vi "Remove.vi"(8 "error in (no error)":errorcluster, 10 "BrowerComponentIDs(\"\")":string[](array[string]), 11 "reference in":refnum<class "BrowerComponent.lvclass">) -> (0 "error out":errorcluster, 3 "reference out":refnum<class "BrowerComponent.lvclass">)   [LabVIEW 2015, in "BrowerComponent.lvclass"]
uses:
  BrowerComponent.lvclass
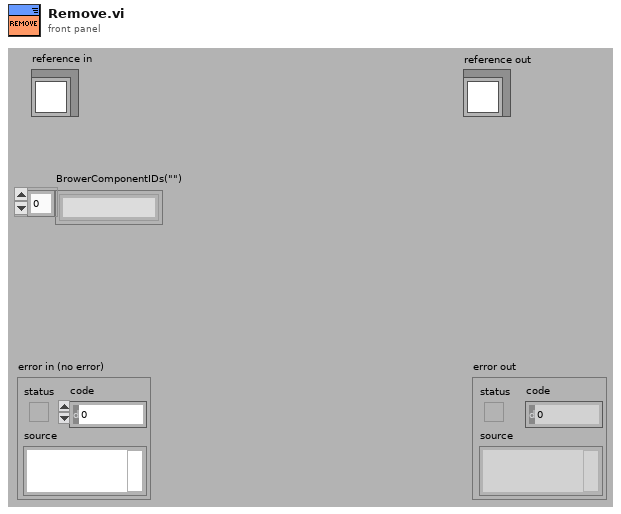
[diagram p1: front panel]
types:
  T1 = typedef "BrowerComponent.lvclass/ObjectAttributes.ctl" = cluster{"ComponentID":string, "SymbolIndex":i32, "ComponentName":string, "PartsOfComponent_dict":variant}
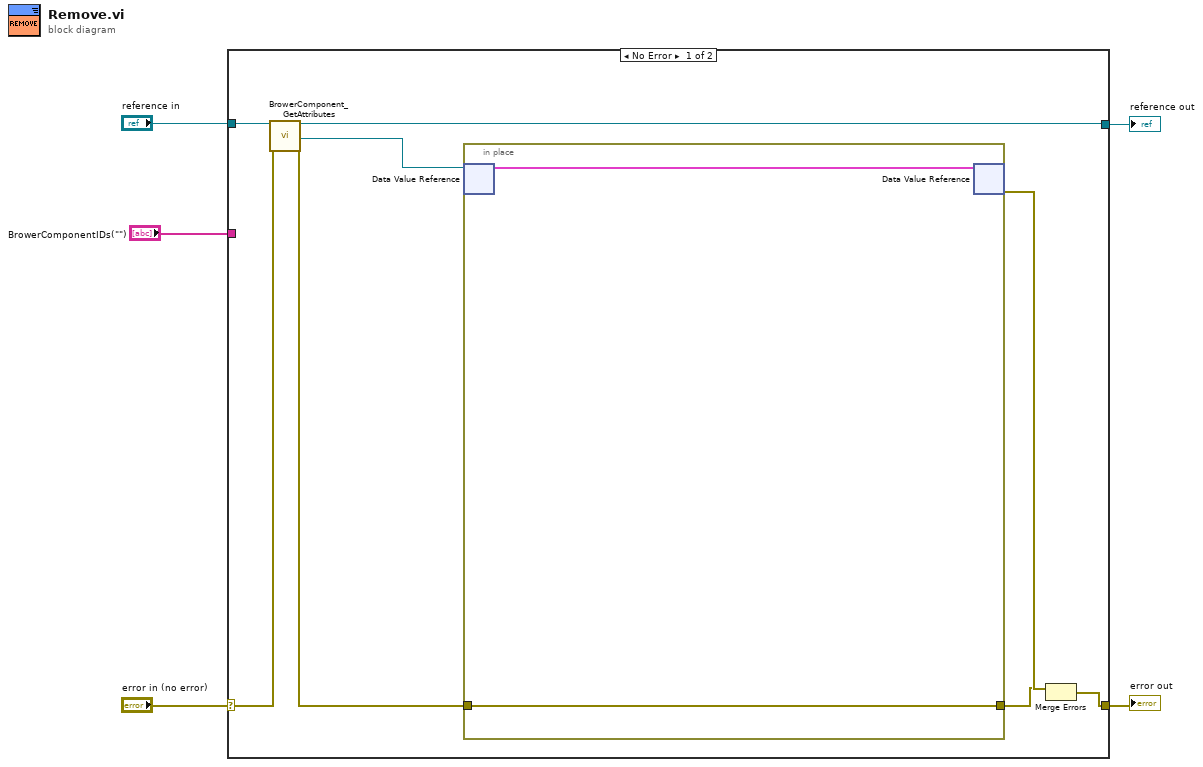
[diagram p0: block diagram]
diagram:
  n1 = case shown="No Error" "error in (no error)" {
    selector: "error in (no error)" -> [w12 w17]
    tunnel: [w9 w17] -> w4
    tunnel: [w10 w16] -> w2
    tunnel: "reference in" -> [w13 w16]
    tunnel: "BrowerComponentIDs(\"\")" -> [_ _]
    frame No Error {
      n2 = call "BrowerComponent_GetAttributes.vi"("reference in"=w13, "error in (no error)"=w12) -> ("reference out"=w10:refnum<class "BrowerComponent.lvclass">, "DataRef"=w8:refnum<data-value>, "error out"=w7:errorcluster)  [unwired: 14 in, 1 out]
      n3 = in-place {
        in-place-border: w7 -> [w14]
        in-place-border: [w14] -> w6
        n4 = in-place-dvr #1(w8) -> (w15:T1)  [unwired: 1 out]
        n5 = in-place-dvr #1(w15) -> (w11:errorcluster)  [unwired: 1 out]
      }
      n6 = Merge Errors(w11, w6) -> (w9:errorcluster)
    }
    frame Error {
    }
  }
  "error out" <- w4
  "reference out" <- w2
